vi "RM.getAllDeviceReservationDBs.vi"(8 "error in":errorcluster, 11 "Item Ref in":T1 format="%.0x") -> (0 "error out":errorcluster, 1 "reservation dbs":variant[](array[variant]), 2 "device names":string[](array[string]), 3 "Item Ref out":T1 format="%.0x", 4 "deviceGUIDs":string[](array[string]))   [LabVIEW 2016, in "FPGA Resource Manager.lvlib"]
uses:
  <vilib>/NI Veristand/Custom Device API/Custom Device Item Ref.ctl
  RM.Globals.vi
  <vilib>/NI Veristand/Custom Device API/Get Item Property (Variant).vi
  <vilib>/NI Veristand/Custom Device API/Get Item Property (String).vi
  FPGA Resource Manager.lvlib
  <vilib>/NI Veristand/Custom Device API/Custom Device API.lvlib
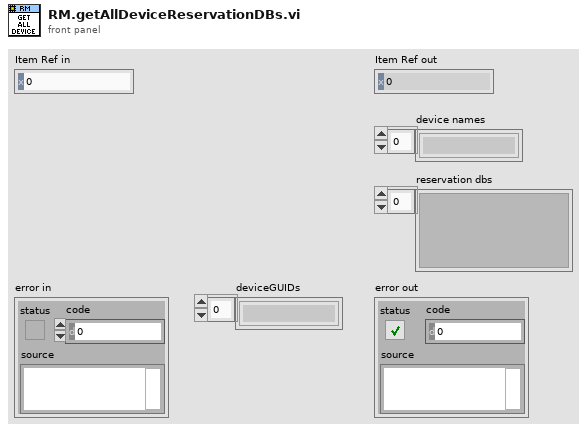
[diagram p1: front panel]
types:
  T1 = typedef "Custom Device API.lvlib/Custom Device Item Ref.ctl" = u64
  T2 = typedef "Custom Device API.lvlib/Custom Device Item Info.ctl" = cluster{"Name":string, "Is Channel":bool, "GUID":string, "Is Waveform":bool}
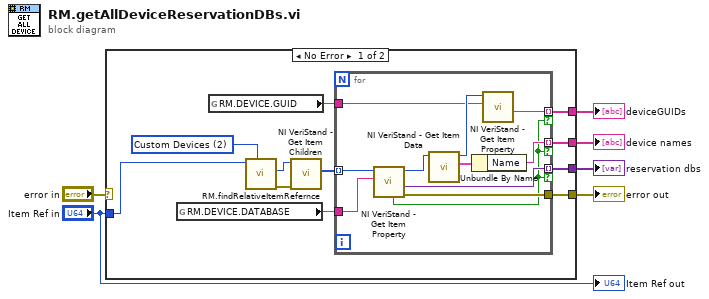
[diagram p0: block diagram]
diagram:
  n1 = case shown="No Error" "error in" {
    selector: "error in" -> [_ w29]
    tunnel: "Item Ref in" -> [w13 _]
    tunnel: [w17 _] -> w3
    tunnel: [w16 _] -> w2
    tunnel: [w15 w29] -> w5
    tunnel: [w9 _] -> w1
    frame No Error {
      w14 = u16 2 items=["Targets", "Controller", "Custom Devices", "This CD", "This CD/Group", "This CD/Group/SubGroup"] ("Relative Type")
      n2 = global read "RM.Globals.vi" "RM.DEVICE.DATABASE"() -> (w8:string)
      n3 = global read "RM.Globals.vi" "RM.DEVICE.GUID"() -> (w7:string)
      n4 = call "RM.findRelativeItemRefernce.vi"("Relative Type"=w14, "Item Ref in"=w13) -> ("error out"=w12:errorcluster, "Relative Item Ref Out"=w11:T1)  [unwired: 5 in, 3 out]
      n5 = call <vilib>:"NI VeriStand - Get Item Children.vi"("error in (no error)"=w12, "Item Ref in"=w11) -> ("Child Refs"=w10:T1[])  [unwired: 6 in, 3 out]
      n6 = for {
        tunnel: w8 -> [w28]
        tunnel: [w22] -> w17 mode=indexing if=w19
        tunnel: [w24] -> w16 mode=indexing if=w19
        tunnel: [w27] -> w15
        tunnel: w10 -> [w26] mode=indexing
        tunnel: [w20] -> w9 mode=indexing if=w19
        tunnel: w7 -> [w18]
        n7 = call-poly <vilib>:"NI VeriStand - Get Item Property.vi"("Property Name"=w28, "Item Ref in"=w26) -> ("error out"=w27:errorcluster, "Value"=w22:variant, "Item Ref out"=w25:T1, "Found?"=w19:bool)  [unwired: 6 in]
        n8 = call <vilib>:"NI VeriStand - Get Item Data.vi"("Item Ref in"=w25) -> ("Item Info"=w23:T2, "Item Ref out"=w21:T1)  [unwired: 7 in, 2 out]
        n9 = Unbundle By Name(w23) -> ("Name"=w24:string)
        n10 = call-poly <vilib>:"NI VeriStand - Get Item Property.vi"("Property Name"=w18, "Item Ref in"=w21) -> ("Value"=w20:string)  [unwired: 6 in, 3 out]
      }
    }
    frame Error {
    }
  }
  "error out" <- w5
  "reservation dbs" <- w3
  "device names" <- w2
  "deviceGUIDs" <- w1
  "Item Ref out" <- "Item Ref in"
